vi "Instances check all.vi"(11 "Array in":string[](array[string])) -> (0 "Any all days?":bool, 3 "Array out":string[](array[string]))   [LabVIEW 2015]
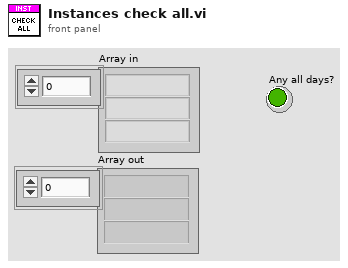
[diagram p1: front panel]
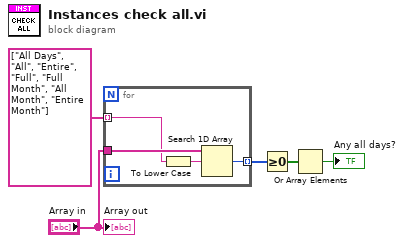
[diagram p0: block diagram]
diagram:
  n1 = for {
    tunnel: "Array in" -> [w9]
    tunnel: string[] ["All Days", "All", "Entire", "Full", "Full Month", "All Month", "Entire Month"] -> [w8] mode=indexing
    tunnel: [w7] -> w3 mode=indexing
    n2 = To Lower Case(string=w8) -> (all lower case string=w6:string)
    n3 = Search 1D Array(1D array=w9, element=w6) -> (index of element=w7:i32)  [unwired: 1 in]
  }
  n4 = Greater Or Equal To 0?(x=w3) -> (x >= 0?=w4:bool[])
  n5 = Or Array Elements(Boolean array=w4) -> (logical OR=→"Any all days?":bool)
  "Array out" <- "Array in"
